vi "Test.vi"   [LabVIEW 2018]
doc: "This VI is called when test mode begins, and will automatically be terminated when it ends. You can add manual or automatic tests and invoke them from the dashboard."
types:
  T1 = typedef "WPI_EncoderDevRef.ctl" = cluster{"DevStatus":errorcluster, "EncoderIndex":T2, "CounterIndex":T3, "DistancePerCount":dbl, "Decoding Type":T4}
  T2 = typedef "FPGA_EncoderIdx.ctl" = enum8{"Enc 0", "Enc 1", "Enc 2", "Enc 3", "Enc 4", "Enc 5", "Enc 6", "Enc 7", "Invalid"}
  T3 = typedef "FPGA_CounterCtrSystemIndex.ctl" = enum8{"Ctr 0", "Ctr 1", "Ctr 2", "Ctr 3", "Ctr 4", "Ctr 5", "Ctr 6", "Ctr 7", "Invalid"}
  T4 = typedef "WPI_EncoderType.ctl" = enum16{"1x", "2x", "4x"}
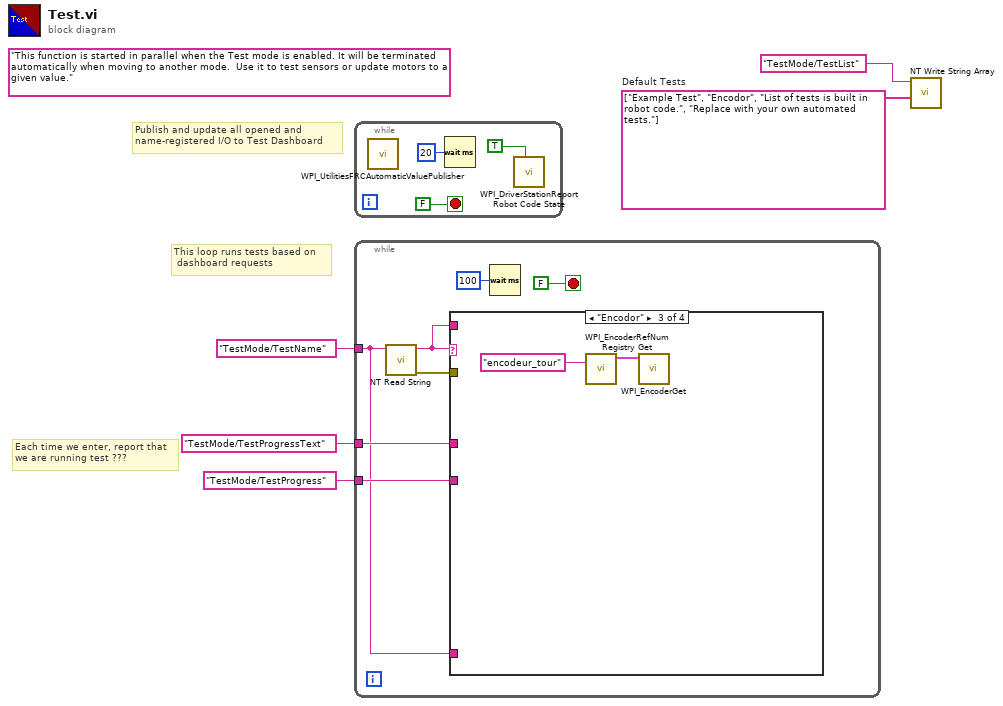
[diagram p0: block diagram]
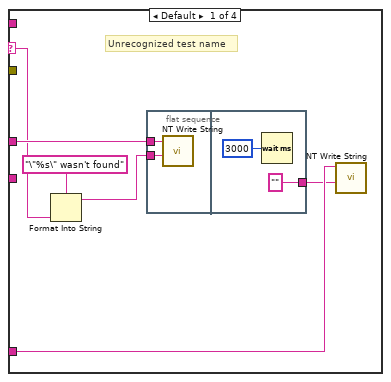
[diagram p2: hidden frame]
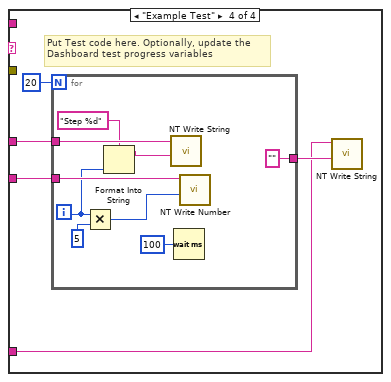
[diagram p4: hidden frame]
diagram:
  w2 = string[] ["Example Test", "Encodor", "List of tests is built in robot code.", "Replace with your own automated tests."]  # Default Tests
  (unwired) "This function is started in parallel when the Test mode is enabled. It will be terminated automatically when moving to another mode.  Use it to test sensors or update motors to a given value."
  # "This loop runs tests based on \n dashboard requests"
  # "Publish and update all opened and\nname-registered I/O to Test Dashboard"
  # "Each time we enter, report that\nwe are running test ???"
  n1 = while {
    stop <- FALSE stop-if-true
    n2 = call <vilib>:"WPI_UtilitiesFRCAutomaticValuePublisher.vi"() -> ()  [unwired: 12 in]
    n3 = Wait (ms)(milliseconds to wait=u32 20) -> ()  [unwired: 1 out]
    n4 = call <vilib>:"WPI_DriverStationReport Robot Code State.vi"("Test"=TRUE ("Autonomous")) -> ()  [unwired: 10 in, 1 out]
  }
  n5 = while {
    tunnel: "TestMode/TestName" ("Name") -> [w10]
    tunnel: "TestMode/TestProgressText" ("Name") -> [w13]
    tunnel: "TestMode/TestProgress" ("Name") -> [w12]
    stop <- FALSE stop-if-true
    n6 = call <vilib>:"NT Read String.vi"("Name"=w10) -> ("error out"=w9:errorcluster, "String"=w11:string)  [unwired: 9 in]
    n7 = case shown="\"Encodor\"" w11 {
      selector: w11 -> [w20 _ _ _]
      tunnel: w10 -> [w17 _ _ w28]
      tunnel: w13 -> [w21 _ _ w31]
      tunnel: w12 -> [_ _ _ w32]
      tunnel: w11 -> [_ _ _ _]
      tunnel: w9 -> [_ _ _ _]
      frame Default {
        # "Unrecognized test name"
        n8 = Format Into String(format string="\"%s\" wasn't found" ("Name"), w20) -> (resulting string=w19:string)  [unwired: 2 in, 1 out]
        n9 = flat-sequence {
          tunnel: w21 -> [w22]
          tunnel: w19 -> [w23]
          tunnel: ["" ("Name")] -> w16
          frame #0 {
            n10 = call <vilib>:"NT Write String.vi"("String"=w23, "Name"=w22) -> ()  [unwired: 9 in, 1 out]
          }
          frame #1 {
            n11 = Wait (ms)(milliseconds to wait=u32 3000) -> ()  [unwired: 1 out]
          }
        }
        n12 = call <vilib>:"NT Write String.vi"("String"=w16, "Name"=w17) -> ()  [unwired: 9 in, 1 out]
      }
      frame "" {
        # "No test to run"
      }
      frame "Encodor" {
        n13 = call <vilib>:"WPI_EncoderRefNum Registry Get.vi"("refnum name"="encodeur_tour" ("Name")) -> ("EncoderDevRef"=w27:T1)  [unwired: 9 in, 1 out]
        n14 = call <vilib>:"WPI_EncoderGet.vi"("EncoderDevRef"=w27) -> ()  [unwired: 5 in, 6 out]
      }
      frame "Example Test" {
        # "Put Test code here. Optionally, update the\nDashboard test progress variables"
        n15 = for {
          N: 20 -> [_]
          tunnel: w32 -> [w41]
          tunnel: w31 -> [w39]
          tunnel: ["" ("String")] -> w29
          i -> [w36]
          n16 = Multiply(x=w36, y=u32 5 ("milliseconds to wait")) -> (x*y=w37:u32)
          n17 = Format Into String(format string="Step %d", w36) -> (resulting string=w34:string)  [unwired: 2 in, 1 out]
          n18 = call <vilib>:"NT Write String.vi"("String"=w34, "Name"=w39) -> ()  [unwired: 9 in, 1 out]
          n19 = Wait (ms)(milliseconds to wait=u32 100) -> ()  [unwired: 1 out]
          n20 = call <vilib>:"NT Write Number.vi"("Numeric"=w37, "Name"=w41) -> ()  [unwired: 9 in, 1 out]
        }
        n21 = call <vilib>:"NT Write String.vi"("String"=w29, "Name"=w28) -> ()  [unwired: 9 in, 1 out]
      }
    }
    n22 = Wait (ms)(milliseconds to wait=u32 100) -> ()  [unwired: 1 out]
  }
  n23 = call <vilib>:"NT Write String Array.vi"("String Array"=w2, "Name"="TestMode/TestList") -> ()  [unwired: 9 in, 1 out]
